vi "Main.vi"   [LabVIEW 2020, in "neg-pkg-cli.lvlib" / "CLI.lvclass"]
uses:
  CLI.lvclass
  CLI.lvclass/CLI.ctl
  MGI Console/Source/Console/Console.lvclass
panel:
  # "CLI\nMain"
types:
  T1 = enum32{"Invalid", "Standard", "Closed", "Hidden", "Minimized", "Maximized"}
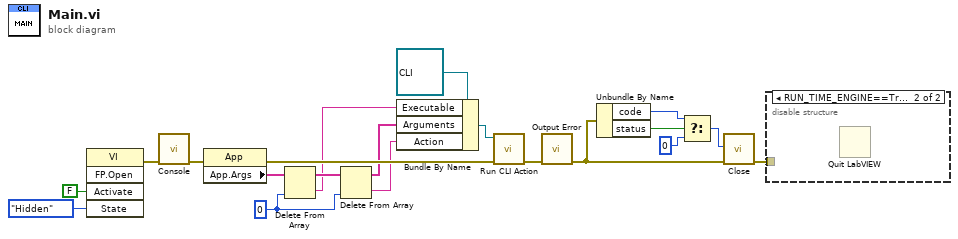
[diagram p0: block diagram]
diagram:
  w17 = 0 ("index")
  n1 = invoke class="VI" method="FP.Open"("Activate"=FALSE ("Activate?"), "State"=T1."Hidden" ("Front Panel Window:State")) -> (error out=w9:errorcluster)  [unwired: 3 in, 4 out]
  n2 = call "Console.vi"("error in (no error)"=w9) -> ("error out"=w1:errorcluster)  [unwired: 10 in]
  n3 = property class="App"(error in=w1) -> (error out=w20:errorcluster, "App.Args"=w19:string[])  [unwired: 1 in, 1 out]
  n4 = Delete From Array(array=w19, index=w17) -> (deleted portion=w15:string, array with subset deleted=w18:string[])  [unwired: 1 in]
  n5 = Delete From Array(array=w18, index=w17) -> (deleted portion=w13:string, array with subset deleted=w14:string[])  [unwired: 1 in]
  n6 = Bundle By Name(cluster=refnum<class "CLI.lvclass"> refnum ("neg-pkg-cli.lvlib:CLI.lvclass"), "Executable"=w15, "Arguments"=w14, "Action"=w13) -> (w12:refnum<class "CLI.lvclass">)
  n7 = call "Run CLI Action.vi"("error in (no error)"=w20, "CLI in"=w12) -> ("error out"=w11:errorcluster)  [unwired: 9 in]
  n8 = call "Output Error.vi"("error in (no error)"=w11) -> ("error out"=w4:errorcluster)  [unwired: 10 in]
  n9 = Unbundle By Name(w4) -> ("code"=w7:i32, "status"=w8:bool)
  n10 = Select(t=w7, s=w8, f=0) -> (s? t:f=w5:i32)
  n11 = call "Close.vi"("error in (no error)"=w4, "Return Code"=w5) -> ("error out"=w3:errorcluster)  [unwired: 9 in]
  n12 = disable-structure shown="RUN_TIME_ENGINE==True" {
    disable-tunnel: w3 -> [_ _]
    frame condition #0 (active) {
    }
    frame condition #1 {
      n13 = Quit LabVIEW() -> ()  [unwired: 1 in]
    }
  }
